vi "Dextra V0.vi"() -> ()   [LabVIEW 2009]
uses:
  <vilib>/Platform/TimedLoop/XDataNode/XDataNode.xnode
  <vilib>/Platform/TimedLoop/XDataNode/loadlvalarms.vi
  <vilib>/Platform/TimedLoop/XDataNode/timing_clust.ctl
  <vilib>/Platform/TimedLoop/XDataNode/nitl_modes.ctl
  <vilib>/Platform/TimedLoop/XDataNode/wakeup.ctl
  <vilib>/Platform/TimedLoop/XDataNode/XDNodeRunTimeDep.lvlib
panel:
  in  "stop":bool
  in  "Tab Control":T1(tab)
  out "Waveform Graph":dynamicdata(graph)
  in  "rate":dbl=1000.0
  in  "number of samples":i32=1000
  in  "Ring 2":u16(ring) items=["Seleccione una opcion", "Grabar archivo", "Leer archivo"]
  out "Waveform Graph 2":dynamicdata(graph)
  out "RMS":dbl
  out "Variance":dbl
  out "Maximum":dbl
  out "Minimum":dbl
  out "Range":dbl
  out "RMS 4":dbl
  out "Variance 4":dbl
  out "Maximum 4":dbl
  out "Minimum 4":dbl
  out "Range 4":dbl
  out "RMS 3":dbl
  out "Variance 3":dbl
  out "Maximum 3":dbl
  out "Minimum 3":dbl
  out "Range 3":dbl
  out "RMS 2":dbl
  out "Variance 2":dbl
  out "Maximum 2":dbl
  out "Minimum 2":dbl
  out "Range 2":dbl
  in  "stop 2":bool
  out "ACM Z":dbl(slide) scale=1.21..2.1
  out "AMC Y":dbl(slide) scale=1.21..2.1
  out "ACM X":dbl(slide) scale=1.21..2.1
  out "ACM X":dbl
  in  "MAX X":dbl
  in  "MIN X":dbl
  out "ACCELEROMETER INPUTS":dynamicdata(graph)
  in  "AMC RATE":dbl=1000.0
  in  "ACM SAMPLES":i32=1000
  out "MAX X-":dbl
  out "MIN X-":dbl
  out "MAX X+":dbl
  out "MIN X+":dbl
  out "X-":bool
  out "X+":bool
  out "X0 2":bool
  in  "X0":dbl
  out "ACM Y":dbl
  in  "MAX Y":dbl
  in  "MIN Y":dbl
  out "MAX Y-":dbl
  out "MIN Y-":dbl
  out "MAX Y+":dbl
  out "MIN Y+":dbl
  out "Y-":bool
  out "Y+":bool
  out "Y0 2":bool
  in  "Y0":dbl
  out "ACM Z":dbl
  in  "MAX Z":dbl
  in  "MIN Z":dbl
  out "MAX Z-":dbl
  out "MIN Z-":dbl
  out "MAX Z+":dbl
  out "MIN Z+":dbl
  out "Z-":bool
  out "Z+":bool
  out "Z0 2":bool
  in  "Z0":dbl
  out "FSR":dynamicdata(graph)
  out "Numeric":dbl
  in  "RATE FSR":dbl=1000.0
  in  "SAMPLES FSR":i32=1000
  in  "Angle Select":dbl
  in  "Ring":u16(ring) items=["Free Run", "Manual"]
  out "Stpfr angle":dbl
  out "Stpfr step":dbl
  out "StpArray":bool[](array[boolean])
  in  "Stpfr Rotation":bool
  in  "Stpfr Run":bool
  in  "Stpfr Speed":dbl(knob) scale=1.0..1000.0
  out "StpArray 2":bool[](array[boolean])
  out "Stpma angle":dbl
  out "Stpma step":dbl
  in  "Stpma Rotation":bool
  in  "Stpma Run":bool
  in  "Stpma Speed":dbl(knob) scale=1.0..1000.0
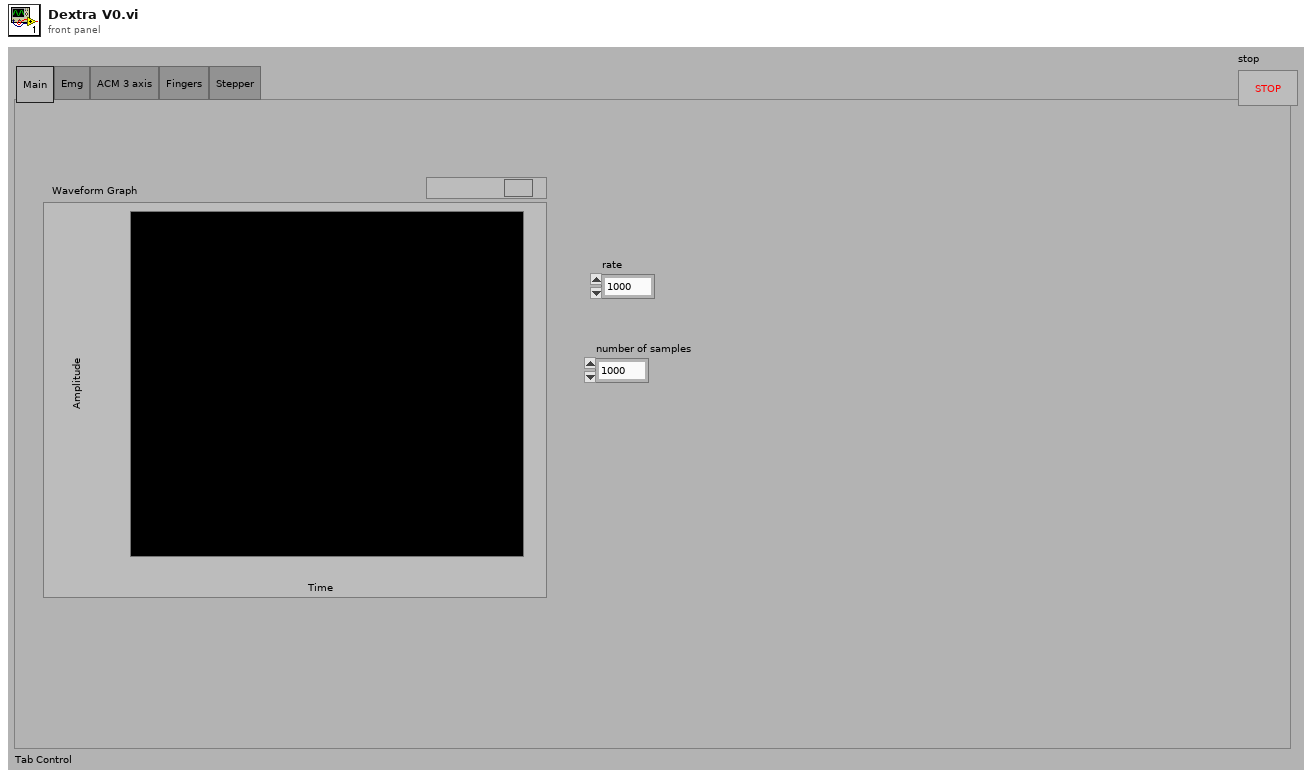
[diagram p1: front panel]
types:
  T1 = enum32{"Main", "Emg", "ACM 3 axis", "Fingers", "Stepper"}
  T2 = typedef "XDNodeRunTimeDep.lvlib/timing_clust.ctl" = cluster{"Expected End [f-1]":u64, "Actual End [f-1]":u64, "Finished Late? [f-1]":bool, "Expected End [i-1]":u64, "Actual End [i-1]":u64, "Finished Late? [i-1]":bool, "Expected Start [i]":u64, "Actual Start [i]":u64, "Expected Start [f]":u64, "Actual Start [f]":u64, "Source Name":string, "Structure Name":string, "Period":i64, "Deadline":i64, "Offset":i64, "Start":i64, "Priority":i32, "Timeout":i32, "Mode":T3, "Wakeup Reason":T4, "Error":errorcluster, "Source Type":string, "Secondary Source Type":string, "Global End Time":u64, "Global Start Time":u64, "Frame Duration":u64, "Iteration Duration":u64, "Assigned CPU":i32, "I/O Scan Engine Mode":u32}
  T3 = typedef "XDNodeRunTimeDep.lvlib/nitl_modes.ctl" = enum32{"No Change", "Process missed periods, maintain original phase", "Discard missed periods, maintain original phase", "Process missed periods, ignore original phase", "Discard missed periods, ignore original phase"}
  T4 = typedef "XDNodeRunTimeDep.lvlib/wakeup.ctl" = enum32{"Normal", "Aborted", "Asynchronous wakeup", "Timing source error", "Timed loop error", "Timeout"}
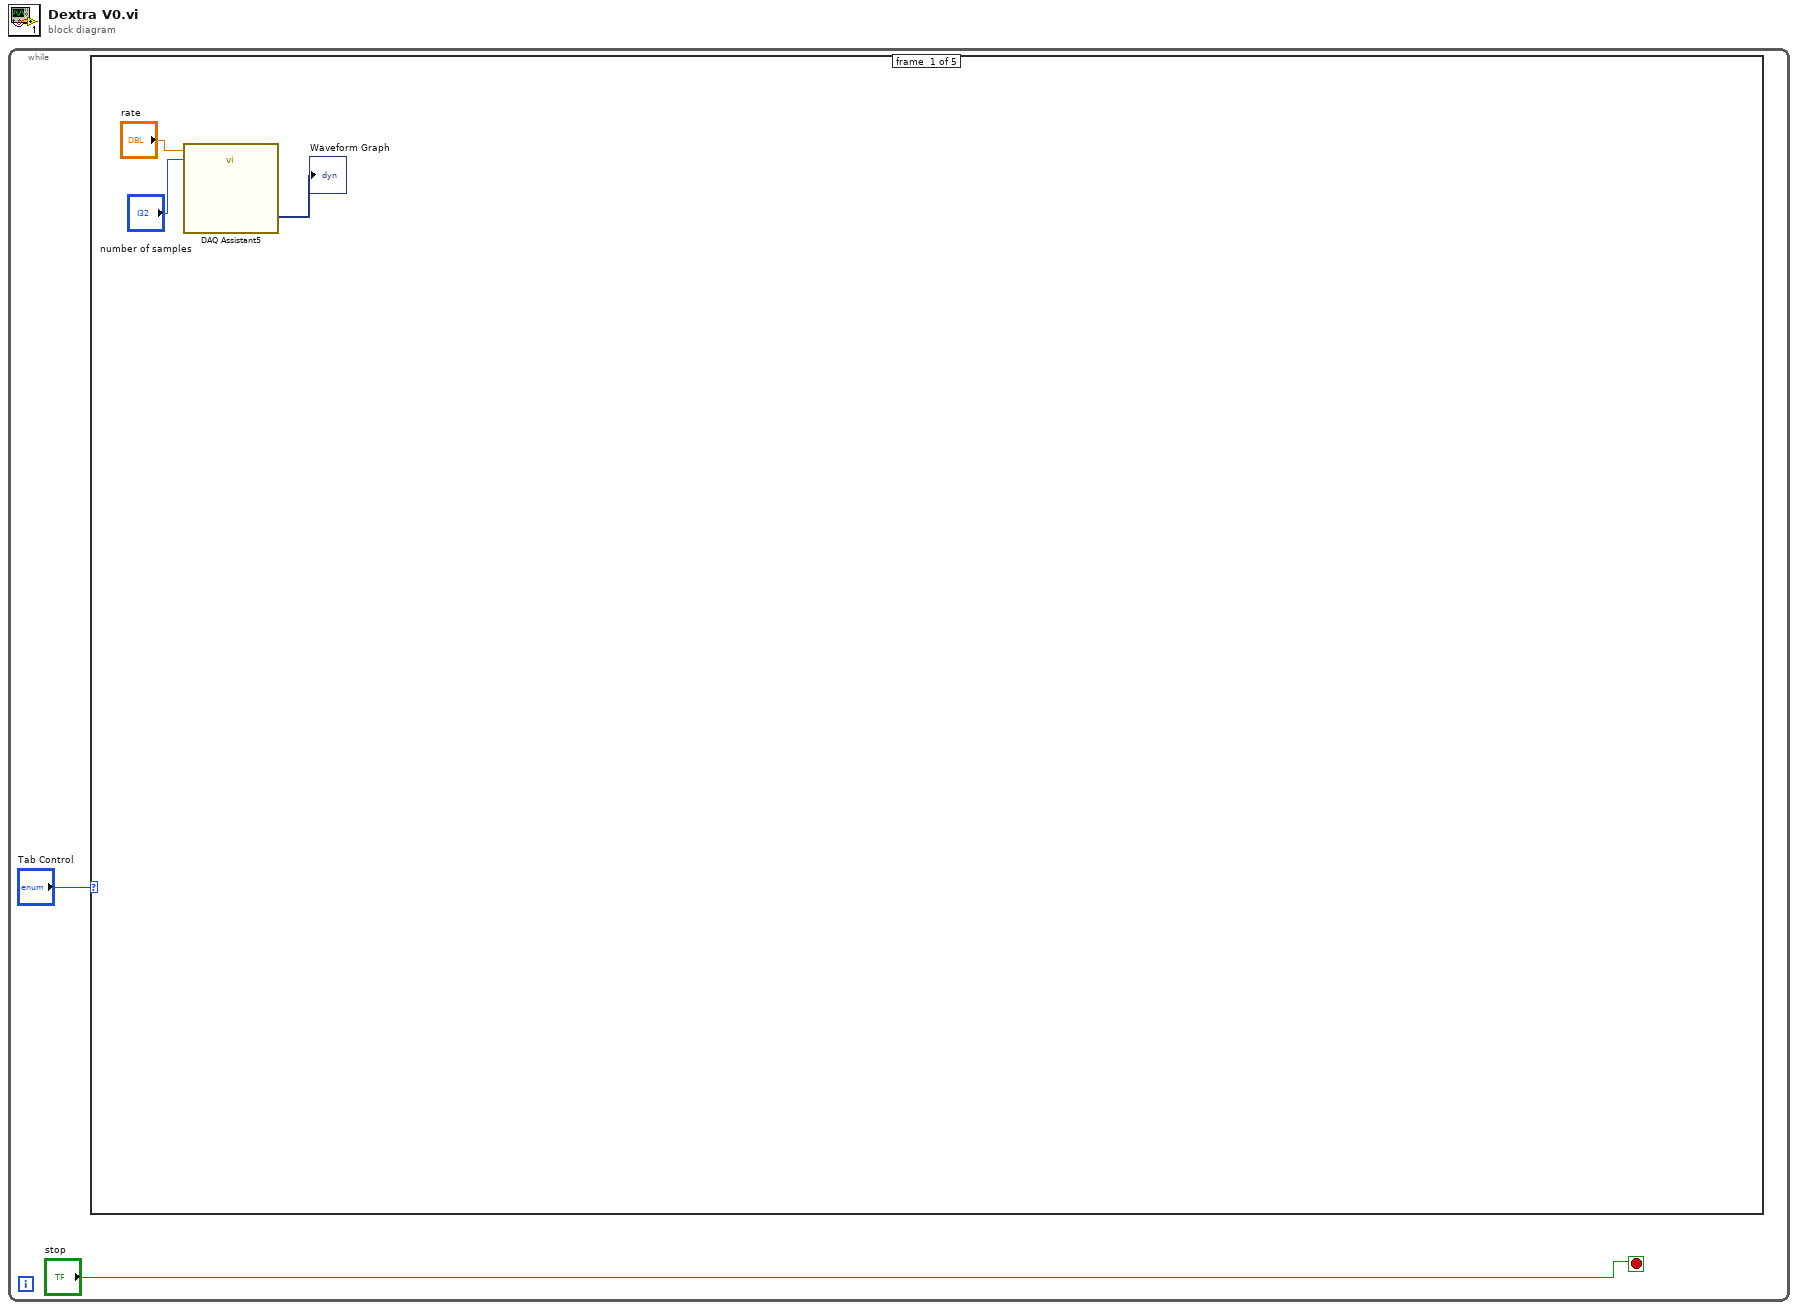
[diagram p0: block diagram]
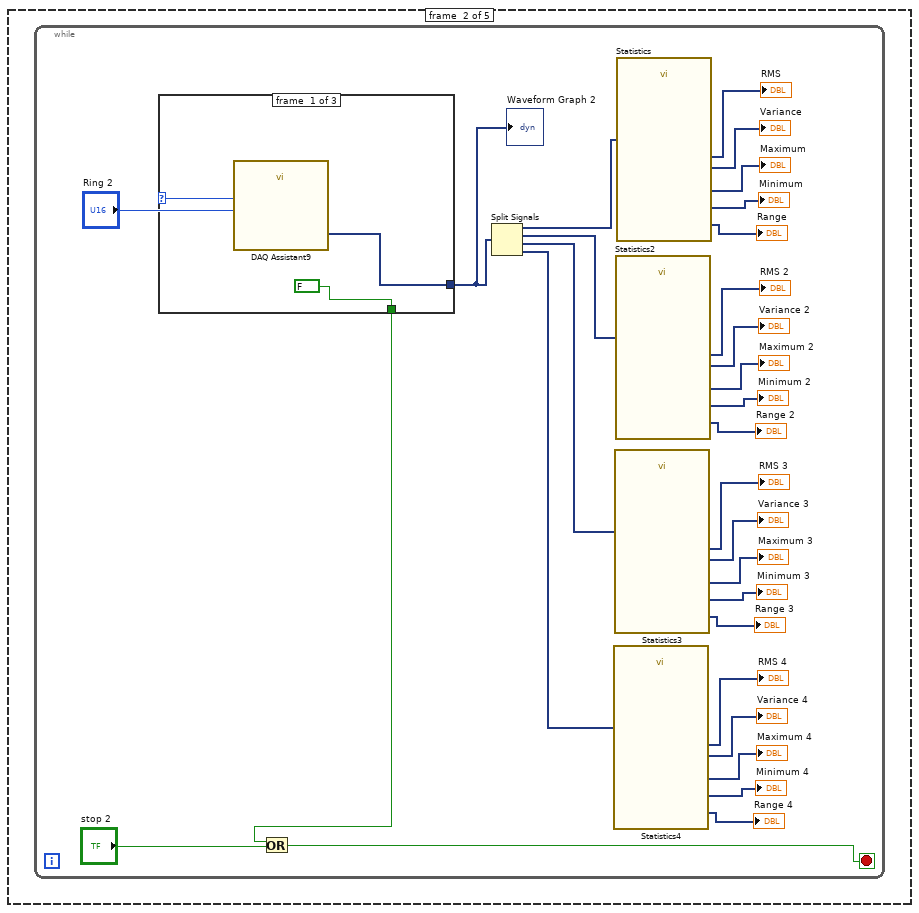
[diagram p2: hidden frame]
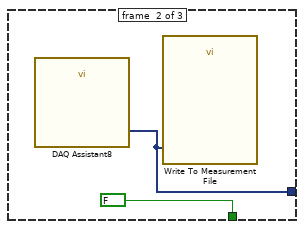
[diagram p3: hidden frame]
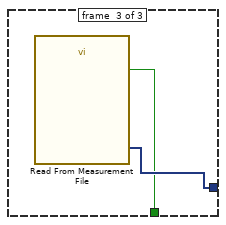
[diagram p4: hidden frame]
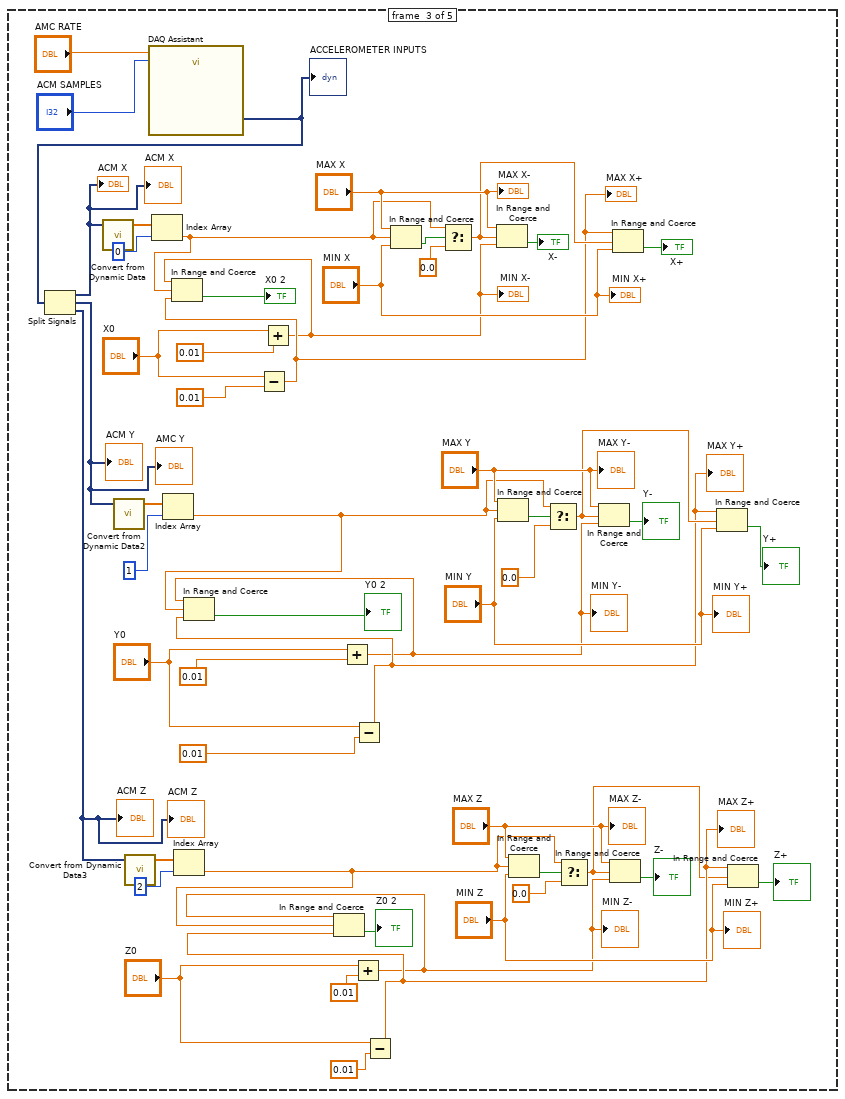
[diagram p5: hidden frame]
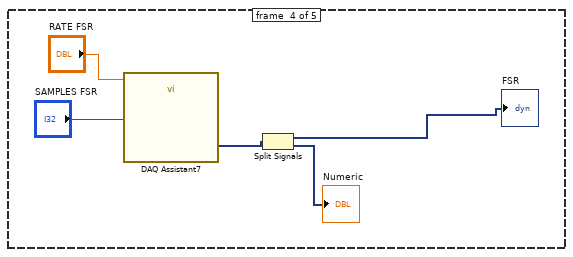
[diagram p6: hidden frame]
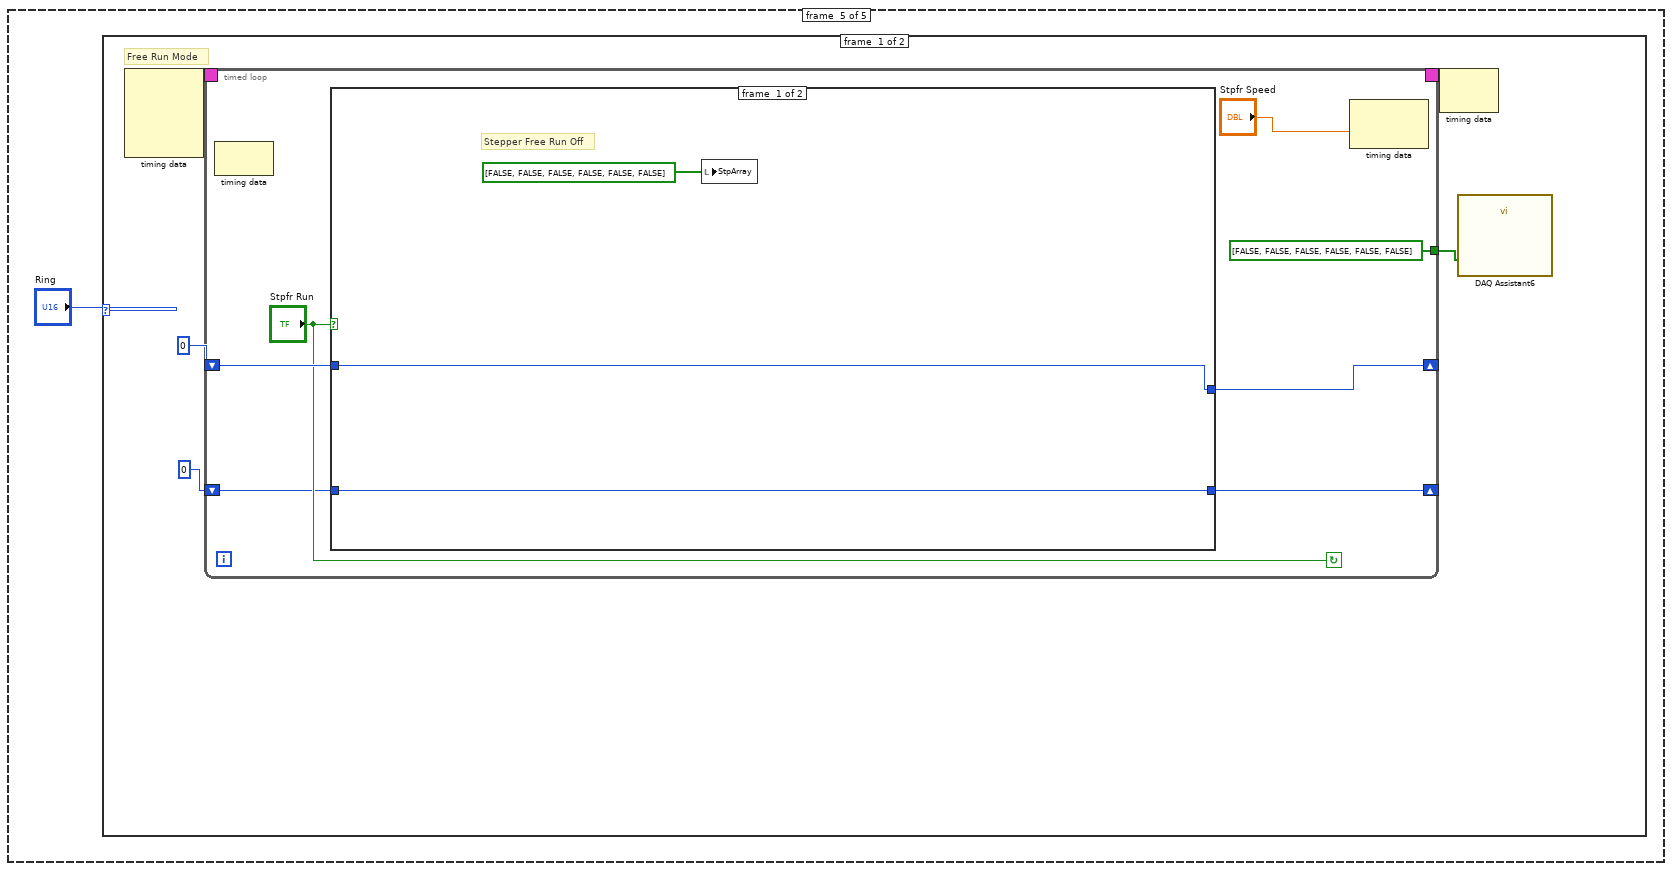
[diagram p7: hidden frame]
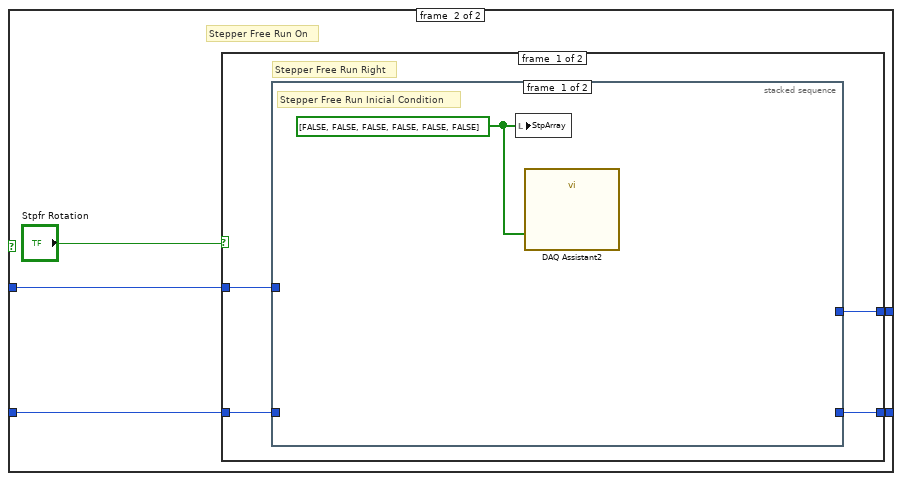
[diagram p8: hidden frame]
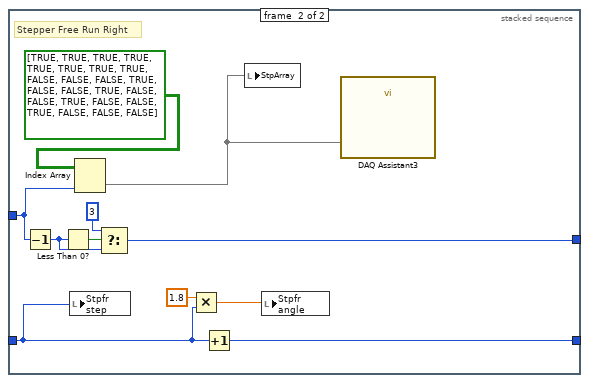
[diagram p9: hidden frame]
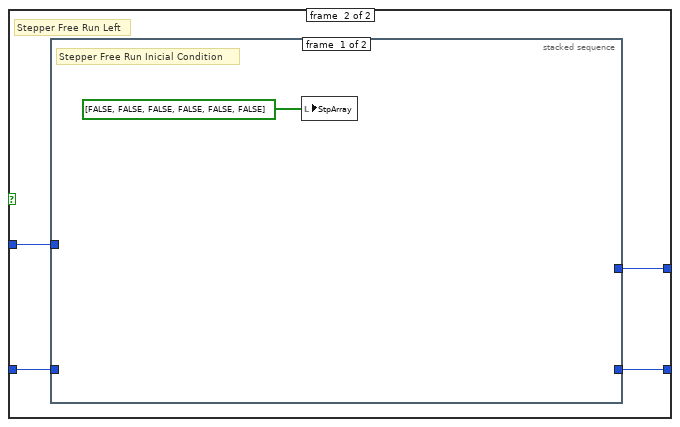
[diagram p10: hidden frame]
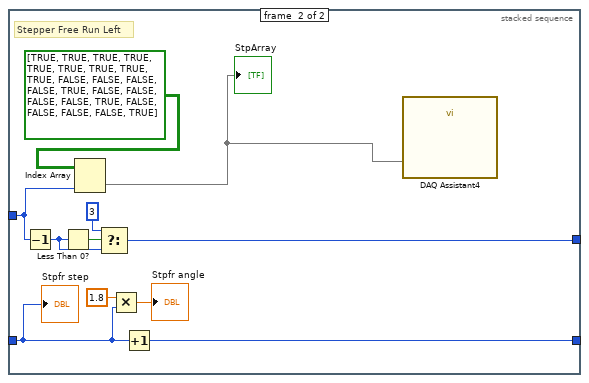
[diagram p11: hidden frame]
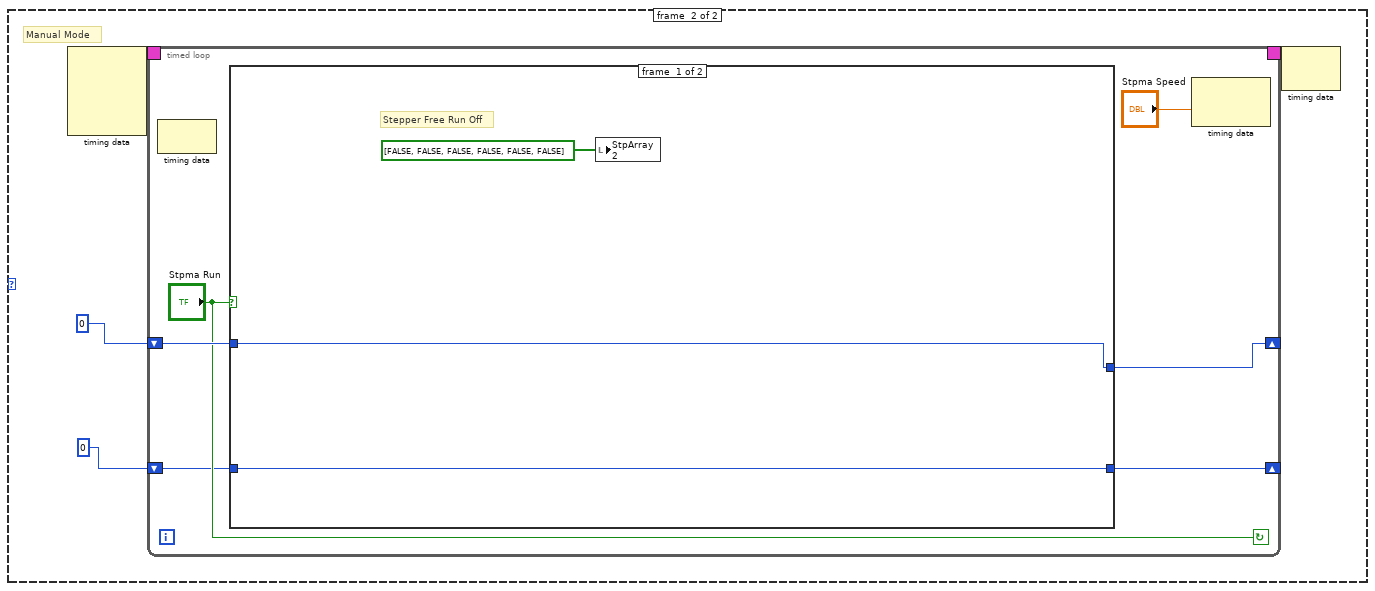
[diagram p12: hidden frame]
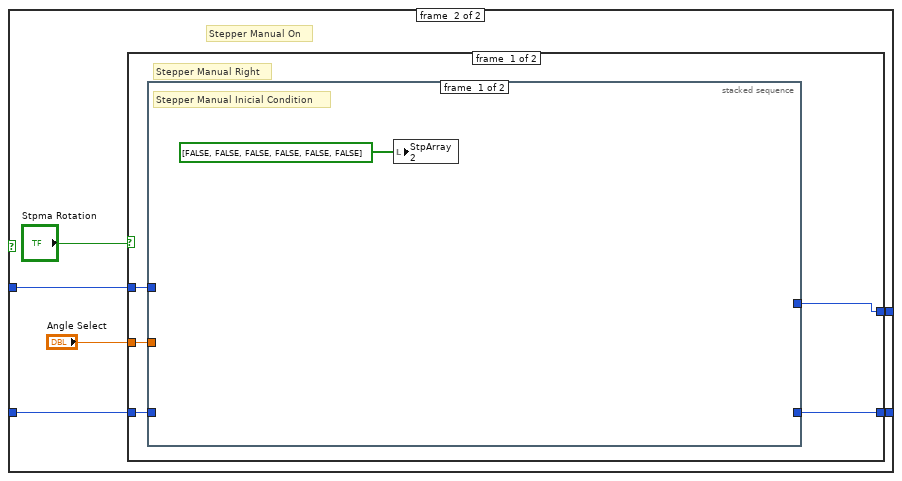
[diagram p13: hidden frame]
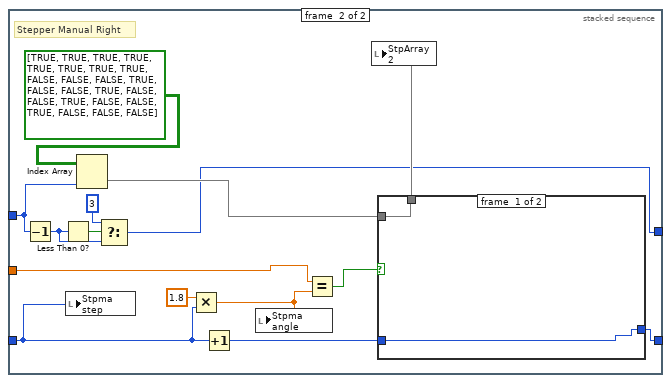
[diagram p14: hidden frame]
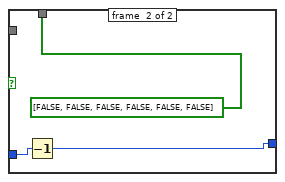
[diagram p15: hidden frame]
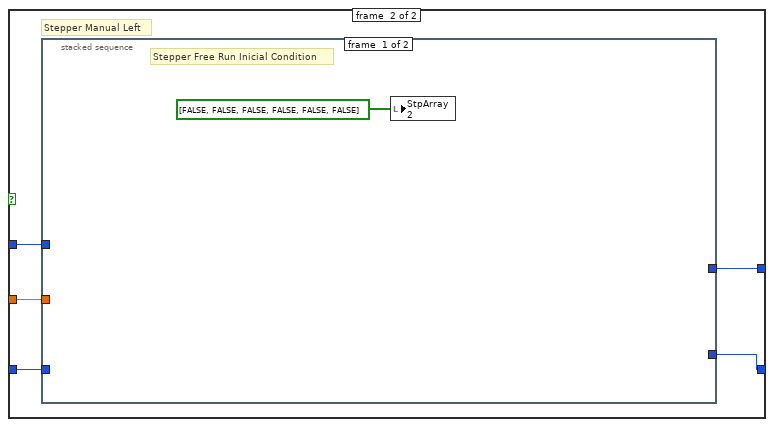
[diagram p16: hidden frame]
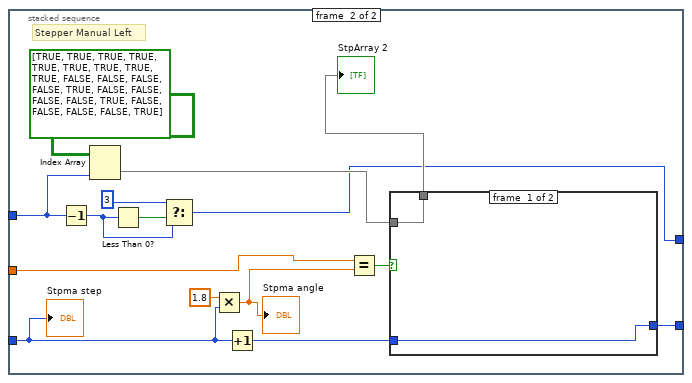
[diagram p17: hidden frame]
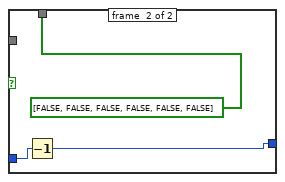
[diagram p18: hidden frame]
diagram:
  n1 = while {
    stop <- "stop" stop-if-true
    n2 = case shown="\"Stepper\"" "Tab Control" {
      frame #0 {
        n3 = call "DAQ Assistant5"("rate"="rate", "number of samples"="number of samples") -> ("data"=→"Waveform Graph":dynamicdata)  [unwired: 15 in, 2 out]
      }
      frame #1 {
        n4 = while {
          stop <- w7 stop-if-true
          n5 = case shown="2" "Ring 2" {
            tunnel: [w36 w38 w40] -> w9
            tunnel: [FALSE FALSE w39] -> w6
            frame #0 {
              n6 = call "DAQ Assistant9"() -> ("data"=w36:dynamicdata)  [unwired: 17 in, 2 out]
            }
            frame #1 {
              n7 = call "DAQ Assistant8"() -> ("data"=w38:dynamicdata)  [unwired: 17 in, 2 out]
              n8 = call "Write To Measurement File"("Signals"=w38) -> ()  [unwired: 16 in, 3 out]
            }
            frame #2 {
              n9 = call "Read From Measurement File"() -> ("Signals"=w40:dynamicdata, "EOF?"=w39:bool)  [unwired: 6 in, 4 out]
            }
          }
          "Waveform Graph 2" <- w9
          n10 = Or(x=w6, y="stop 2") -> (x .or. y?=w7:bool)
          n11 = Split Signals(w9) -> (w14:dynamicdata, w13:dynamicdata, w12:dynamicdata, w11:dynamicdata)  [unwired: 4 in]
          n12 = call "Statistics4"("Signals"=w11) -> ("Variance"=→"Variance 4":dynamicdata, "RMS"=→"RMS 4":dynamicdata, "Range"=→"Range 4":dynamicdata, "Minimum"=→"Minimum 4":dynamicdata, "Maximum"=→"Maximum 4":dynamicdata)  [unwired: 21 in, 1 out]
          n13 = call "Statistics3"("Signals"=w12) -> ("Variance"=→"Variance 3":dynamicdata, "RMS"=→"RMS 3":dynamicdata, "Range"=→"Range 3":dynamicdata, "Minimum"=→"Minimum 3":dynamicdata, "Maximum"=→"Maximum 3":dynamicdata)  [unwired: 21 in, 1 out]
          n14 = call "Statistics2"("Signals"=w13) -> ("Variance"=→"Variance 2":dynamicdata, "RMS"=→"RMS 2":dynamicdata, "Range"=→"Range 2":dynamicdata, "Minimum"=→"Minimum 2":dynamicdata, "Maximum"=→"Maximum 2":dynamicdata)  [unwired: 21 in, 1 out]
          n15 = call "Statistics"("Signals"=w14) -> ("Variance"=→"Variance":dynamicdata, "RMS"=→"RMS":dynamicdata, "Range"=→"Range":dynamicdata, "Minimum"=→"Minimum":dynamicdata, "Maximum"=→"Maximum":dynamicdata)  [unwired: 21 in, 1 out]
        }
      }
      frame #2 {
        n16 = call "DAQ Assistant"("rate"="AMC RATE", "number of samples"="ACM SAMPLES") -> ("data"=w44:dynamicdata)  [unwired: 15 in, 2 out]
        "ACCELEROMETER INPUTS" <- w44
        n17 = Split Signals(w44) -> (w42:dynamicdata, w41:dynamicdata, w43:dynamicdata)  [unwired: 3 in]
        "ACM X" <- w42
        "ACM Y" <- w41
        "ACM Z" <- w43
        "ACM X" <- w42
        "AMC Y" <- w41
        "ACM Z" <- w43
        n18 = call "Convert from Dynamic Data"("Dynamic Data Type"=w42) -> ("Array"=w92:dbl[])  [unwired: 3 in]
        n19 = call "Convert from Dynamic Data2"("Dynamic Data Type"=w41) -> ("Array"=w76:dbl[])  [unwired: 3 in]
        n20 = call "Convert from Dynamic Data3"("Dynamic Data Type"=w43) -> ("Array"=w60:dbl[])  [unwired: 3 in]
        n21 = Index Array(array=w92, index=0) -> (element=w79:dbl)
        n22 = Index Array(array=w76, index=1) -> (element=w63:dbl)
        n23 = Index Array(array=w60, index=2) -> (element=w48:dbl)
        n24 = Subtract(x="X0", y=0.01) -> (x-y=w78:dbl)
        "MAX X+" <- w78
        n25 = Add(x="X0", y=0.01) -> (x+y=w77:dbl)
        "MIN X-" <- w77
        n26 = In Range and Coerce(upper limit=w77, x=w79, lower limit=w78) -> (In Range?=→"X0 2":bool)  [unwired: 1 out]
        n27 = Add(x="Y0", y=0.01) -> (x+y=w61:dbl)
        "MIN Y-" <- w61
        n28 = Add(x="Z0", y=0.01) -> (x+y=w46:dbl)
        "MIN Z-" <- w46
        n29 = Subtract(x="Y0", y=0.01) -> (x-y=w62:dbl)
        "MAX Y+" <- w62
        n30 = In Range and Coerce(upper limit=w61, x=w63, lower limit=w62) -> (In Range?=→"Y0 2":bool)  [unwired: 1 out]
        n31 = Subtract(x="Z0", y=0.01) -> (x-y=w47:dbl)
        "MAX Z+" <- w47
        n32 = In Range and Coerce(upper limit=w46, x=w48, lower limit=w47) -> (In Range?=→"Z0 2":bool)  [unwired: 1 out]
        n33 = In Range and Coerce(upper limit="MAX X", x=w79, lower limit="MIN X") -> (In Range?=w90:bool)  [unwired: 1 out]
        n34 = Select(t=w79, s=w90, f=0.0) -> (s? t:f=w86:dbl)
        n35 = In Range and Coerce(upper limit="MAX X", x=w86, lower limit=w77) -> (In Range?=→"X-":bool)  [unwired: 1 out]
        n36 = In Range and Coerce(upper limit="MAX Y", x=w63, lower limit="MIN Y") -> (In Range?=w74:bool)  [unwired: 1 out]
        n37 = In Range and Coerce(upper limit="MAX Z", x=w48, lower limit="MIN Z") -> (In Range?=w58:bool)  [unwired: 1 out]
        n38 = Select(t=w63, s=w74, f=0.0) -> (s? t:f=w70:dbl)
        n39 = Select(t=w48, s=w58, f=0.0) -> (s? t:f=w45:dbl)
        n40 = In Range and Coerce(upper limit="MAX Y", x=w70, lower limit=w61) -> (In Range?=→"Y-":bool)  [unwired: 1 out]
        n41 = In Range and Coerce(upper limit="MAX Z", x=w45, lower limit=w46) -> (In Range?=→"Z-":bool)  [unwired: 1 out]
        n42 = In Range and Coerce(upper limit=w78, x=w86, lower limit="MIN X") -> (In Range?=→"X+":bool)  [unwired: 1 out]
        n43 = In Range and Coerce(upper limit=w62, x=w70, lower limit="MIN Y") -> (In Range?=→"Y+":bool)  [unwired: 1 out]
        n44 = In Range and Coerce(upper limit=w47, x=w45, lower limit="MIN Z") -> (In Range?=→"Z+":bool)  [unwired: 1 out]
        "MAX X-" <- "MAX X"
        "MIN X+" <- "MIN X"
        "MAX Y-" <- "MAX Y"
        "MIN Y+" <- "MIN Y"
        "MAX Z-" <- "MAX Z"
        "MIN Z+" <- "MIN Z"
      }
      frame #3 {
        n45 = call "DAQ Assistant7"("rate"="RATE FSR", "number of samples"="SAMPLES FSR") -> ("data"=w97:dynamicdata)  [unwired: 15 in, 2 out]
        n46 = Split Signals(w97) -> (→"FSR":dynamicdata, →"Numeric":dynamicdata)  [unwired: 2 in]
      }
      frame #4 {
        n47 = case shown="0, Default" "Ring" {
          frame #0 {
            # "Free Run Mode"
            n48 = node-c288() -> (w105:T2)  [unwired: 4 in]
            n49 = timed-loop {
              timing: w105 -> [_]
              timing-out: [_] -> w104
              shift-right: [w110] -> _
              shift-left: 0 -> [w111]
              shift-right: [w107] -> _
              shift-left: 0 -> [w108]
              tunnel: [bool[] [FALSE, FALSE, FALSE, FALSE, FALSE, FALSE]] -> w101
              stop <- "Stpfr Run" continue-if-true
              n50 = node-c288() -> ()  [unwired: 1 in, 1 out]
              n51 = case shown="True" "Stpfr Run" {
                tunnel: w111 -> [w114 w119]
                tunnel: [w114 w118] -> w110
                tunnel: w108 -> [w113 w117]
                tunnel: [w113 w116] -> w107
                frame #0 {
                  # "Stepper Free Run Off"
                  n52 = local write "StpArray"(bool[] [FALSE, FALSE, FALSE, FALSE, FALSE, FALSE]) -> ()
                }
                frame #1 {
                  # "Stepper Free Run On"
                  n53 = case shown="True" "Stpfr Rotation" {
                    tunnel: w119 -> [w124 w140]
                    tunnel: [w121 w139] -> w118
                    tunnel: w117 -> [w123 w138]
                    tunnel: [w122 w137] -> w116
                    frame #0 {
                      # "Stepper Free Run Right"
                      n54 = stacked-sequence {
                        tunnel: w124 -> [_ w131]
                        tunnel: [_ w132] -> w121
                        tunnel: w123 -> [_ w128]
                        tunnel: [_ w130] -> w122
                        frame #0 {
                          w125 = bool[] [FALSE, FALSE, FALSE, FALSE, FALSE, FALSE]
                          # "Stepper Free Run Inicial Condition"
                          n55 = local write "StpArray"(w125) -> ()
                          n56 = call "DAQ Assistant2"("data"=w125) -> ()  [unwired: 17 in, 2 out]
                        }
                        frame #1 {
                          # "Stepper Free Run Right"
                          n57 = Decrement(x=w131) -> (x-1=w133:i32)
                          n58 = Less Than 0?(x=w133) -> (x < 0?=w135:bool)
                          n59 = local write "Stpfr step"(w128) -> ()
                          n60 = Index Array(array=bool[][] [[TRUE, TRUE, TRUE, TRUE], [TRUE, TRUE, TRUE, TRUE], [FALSE, FALSE, FALSE, TRUE], [FALSE, FALSE, TRUE, FALSE], [FALSE, TRUE, FALSE, FALSE], [TRUE, FALSE, FALSE, FALSE]], index (col)=w131) -> (element=w126:bool[])  [unwired: 1 in]
                          n61 = Select(t=3, s=w135, f=w133) -> (s? t:f=w132:i32)
                          n62 = Multiply(x=1.8, y=w128) -> (x*y=w127:dbl)
                          n63 = Increment(x=w128) -> (x+1=w130:i32)
                          n64 = local write "StpArray"(w126) -> ()
                          n65 = local write "Stpfr angle"(w127) -> ()
                          n66 = call "DAQ Assistant3"("data"=w126) -> ()  [unwired: 17 in, 2 out]
                        }
                      }
                    }
                    frame #1 {
                      # "Stepper Free Run Left"
                      n67 = stacked-sequence {
                        tunnel: w140 -> [_ w147]
                        tunnel: [_ w148] -> w139
                        tunnel: w138 -> [_ w144]
                        tunnel: [_ w146] -> w137
                        frame #0 {
                          # "Stepper Free Run Inicial Condition"
                          n68 = local write "StpArray"(bool[] [FALSE, FALSE, FALSE, FALSE, FALSE, FALSE]) -> ()
                        }
                        frame #1 {
                          # "Stepper Free Run Left"
                          n69 = Decrement(x=w147) -> (x-1=w149:i32)
                          n70 = Less Than 0?(x=w149) -> (x < 0?=w151:bool)
                          n71 = Index Array(array=bool[][] [[TRUE, TRUE, TRUE, TRUE], [TRUE, TRUE, TRUE, TRUE], [TRUE, FALSE, FALSE, FALSE], [FALSE, TRUE, FALSE, FALSE], [FALSE, FALSE, TRUE, FALSE], [FALSE, FALSE, FALSE, TRUE]], index (col)=w147) -> (element=w142:bool[])  [unwired: 1 in]
                          "StpArray" <- w142
                          n72 = Select(t=3, s=w151, f=w149) -> (s? t:f=w148:i32)
                          n73 = Multiply(x=1.8, y=w144) -> (x*y=→"Stpfr angle":dbl)
                          n74 = Increment(x=w144) -> (x+1=w146:i32)
                          n75 = call "DAQ Assistant4"("data"=w142) -> ()  [unwired: 17 in, 2 out]
                          "Stpfr step" <- w144
                        }
                      }
                    }
                  }
                }
              }
              n76 = node-c288("Stpfr Speed") -> ()  [unwired: 1 in, 1 out]
            }
            n77 = node-c288(w104) -> ()  [unwired: 1 out]
            n78 = call "DAQ Assistant6"("data"=w101) -> ()  [unwired: 17 in, 2 out]
          }
          frame #1 {
            # "Manual Mode"
            n79 = node-c288() -> (w162:T2)  [unwired: 4 in]
            n80 = timed-loop {
              timing: w162 -> [_]
              timing-out: [_] -> w161
              shift-right: [w166] -> _
              shift-left: 0 -> [w167]
              shift-right: [w163] -> _
              shift-left: 0 -> [w164]
              stop <- "Stpma Run" continue-if-true
              n81 = node-c288() -> ()  [unwired: 1 in, 1 out]
              n82 = case shown="True" "Stpma Run" {
                tunnel: w167 -> [w170 w176]
                tunnel: [w170 w175] -> w166
                tunnel: w164 -> [w169 w174]
                tunnel: [w169 w173] -> w163
                frame #0 {
                  # "Stepper Free Run Off"
                  n83 = local write "StpArray 2"(bool[] [FALSE, FALSE, FALSE, FALSE, FALSE, FALSE]) -> ()
                }
                frame #1 {
                  # "Stepper Manual On"
                  n84 = case shown="True" "Stpma Rotation" {
                    tunnel: w176 -> [w182 w208]
                    tunnel: [w179 w205] -> w175
                    tunnel: w174 -> [w181 w207]
                    tunnel: [w180 w206] -> w173
                    tunnel: "Angle Select" -> [w178 w204]
                    frame #0 {
                      # "Stepper Manual Right"
                      n85 = stacked-sequence {
                        tunnel: w182 -> [_ w194]
                        tunnel: w181 -> [_ w192]
                        tunnel: [_ w186] -> w180
                        tunnel: [_ w185] -> w179
                        tunnel: w178 -> [_ w184]
                        frame #0 {
                          # "Stepper Manual Inicial Condition"
                          n86 = local write "StpArray 2"(bool[] [FALSE, FALSE, FALSE, FALSE, FALSE, FALSE]) -> ()
                        }
                        frame #1 {
                          # "Stepper Manual Right"
                          n87 = Decrement(x=w194) -> (x-1=w195:i32)
                          n88 = Less Than 0?(x=w195) -> (x < 0?=w197:bool)
                          n89 = local write "Stpma step"(w192) -> ()
                          n90 = Index Array(array=bool[][] [[TRUE, TRUE, TRUE, TRUE], [TRUE, TRUE, TRUE, TRUE], [FALSE, FALSE, FALSE, TRUE], [FALSE, FALSE, TRUE, FALSE], [FALSE, TRUE, FALSE, FALSE], [TRUE, FALSE, FALSE, FALSE]], index (col)=w194) -> (element=w188:bool[])  [unwired: 1 in]
                          n91 = Select(t=3, s=w197, f=w195) -> (s? t:f=w185:i32)
                          n92 = Multiply(x=1.8, y=w192) -> (x*y=w191:dbl)
                          n93 = Increment(x=w192) -> (x+1=w187:i32)
                          n94 = local write "Stpma angle"(w191) -> ()
                          n95 = Equal?(x=w184, y=w191) -> (x = y?=w190:bool)
                          n96 = case shown="False" w190 {
                            tunnel: [w200 bool[] [FALSE, FALSE, FALSE, FALSE, FALSE, FALSE]] -> w189
                            tunnel: w188 -> [w200 _]
                            tunnel: w187 -> [w199 w202]
                            tunnel: [w199 w201] -> w186
                            frame #0 {
                            }
                            frame #1 {
                              n97 = Decrement(x=w202) -> (x-1=w201:i32)
                            }
                          }
                          n98 = local write "StpArray 2"(w189) -> ()
                        }
                      }
                    }
                    frame #1 {
                      # "Stepper Manual Left"
                      n99 = stacked-sequence {
                        tunnel: w208 -> [_ w220]
                        tunnel: w207 -> [_ w219]
                        tunnel: [_ w214] -> w206
                        tunnel: [_ w213] -> w205
                        tunnel: w204 -> [_ w210]
                        frame #0 {
                          # "Stepper Free Run Inicial Condition"
                          n100 = local write "StpArray 2"(bool[] [FALSE, FALSE, FALSE, FALSE, FALSE, FALSE]) -> ()
                        }
                        frame #1 {
                          # "Stepper Manual Left"
                          n101 = Decrement(x=w220) -> (x-1=w221:i32)
                          n102 = Index Array(array=bool[][] [[TRUE, TRUE, TRUE, TRUE], [TRUE, TRUE, TRUE, TRUE], [TRUE, FALSE, FALSE, FALSE], [FALSE, TRUE, FALSE, FALSE], [FALSE, FALSE, TRUE, FALSE], [FALSE, FALSE, FALSE, TRUE]], index (col)=w220) -> (element=w217:bool[])  [unwired: 1 in]
                          n103 = Less Than 0?(x=w221) -> (x < 0?=w223:bool)
                          n104 = Select(t=3, s=w223, f=w221) -> (s? t:f=w213:i32)
                          n105 = Multiply(x=1.8, y=w219) -> (x*y=w211:dbl)
                          "Stpma angle" <- w211
                          n106 = Increment(x=w219) -> (x+1=w215:i32)
                          n107 = Equal?(x=w210, y=w211) -> (x = y?=w212:bool)
                          n108 = case shown="False" w212 {
                            tunnel: [w226 bool[] [FALSE, FALSE, FALSE, FALSE, FALSE, FALSE]] -> w216
                            tunnel: [w225 w228] -> w214
                            tunnel: w217 -> [w226 _]
                            tunnel: w215 -> [w225 w227]
                            frame #0 {
                            }
                            frame #1 {
                              n109 = Decrement(x=w227) -> (x-1=w228:i32)
                            }
                          }
                          "StpArray 2" <- w216
                          "Stpma step" <- w219
                        }
                      }
                    }
                  }
                }
              }
              n110 = node-c288("Stpma Speed") -> ()  [unwired: 1 in, 1 out]
            }
            n111 = node-c288(w161) -> ()  [unwired: 1 out]
          }
        }
      }
    }
  }
